vi "GetRange.vi"(11 "String":string) -> (0 "#Col Elements":i32, 1 "Start Column":i32, 2 "#RowElements":i32, 3 "Start Row":i32)   [LabVIEW 2014]
panel:
  # "Input"
  # "Output"
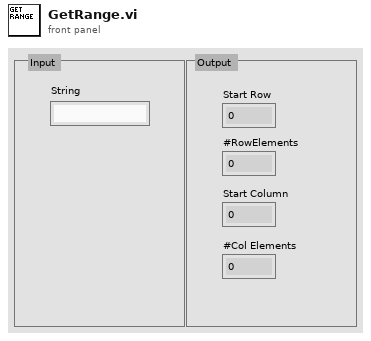
[diagram p1: front panel]
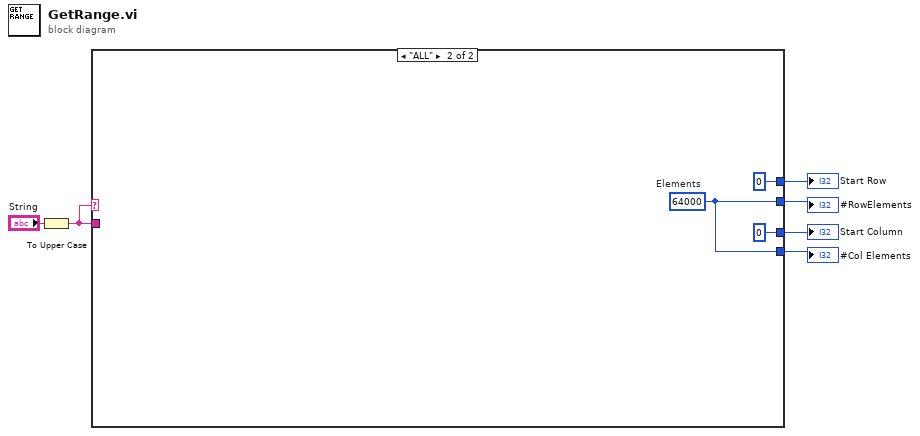
[diagram p0: block diagram]
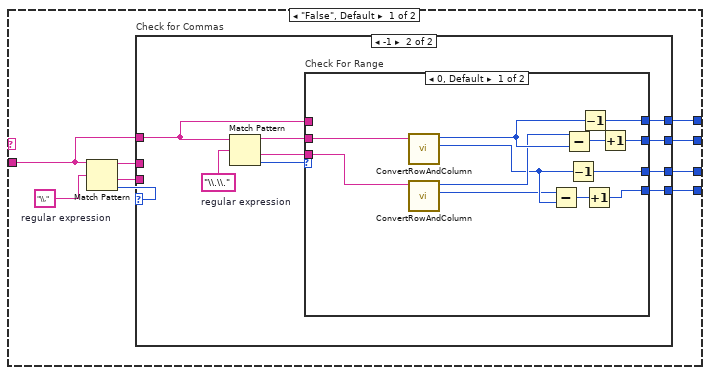
[diagram p2: hidden frame]
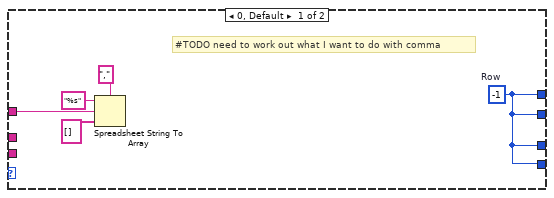
[diagram p3: hidden frame]
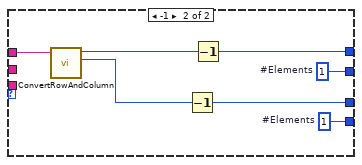
[diagram p4: hidden frame]
diagram:
  n1 = To Upper Case(1:"String") -> (0:w1:string)
  n2 = case shown="\"ALL\"" w1 {
    tunnel: [w11 0 ("Row")] -> w5
    tunnel: [w10 w49] -> w4
    tunnel: [w9 0 ("Row")] -> w3
    tunnel: [w8 w49] -> w2
    tunnel: w1 -> [w7 _]
    frame "False", Default {
      w12 = "\\,"  # regular expression
      n3 = Match Pattern(string=w7, regular expression=w12) -> (before substring=w14:string, after substring=w13:string, offset past match=w15:i32)  [unwired: 1 in, 1 out]
      n4 = case "Check for Commas" shown="-1" w15 {
        tunnel: w14 -> [_ _]
        tunnel: w13 -> [_ _]
        tunnel: w7 -> [w19 w25]
        tunnel: [w16 w24] -> w11
        tunnel: [w16 w23] -> w10
        tunnel: [w16 w22] -> w9
        tunnel: [w16 w21] -> w8
        frame 0, Default {
          w16 = -1  # Row
          # "#TODO need to work out what I want to do with comma"
          n5 = Spreadsheet String To Array(delimiter (Tab)=",", format string="%s", spreadsheet string=w19, array type (2D Dbl)=string[] []) -> ()  [unwired: 1 out]
        }
        frame -1 {
          w29 = "\\.\\."  # regular expression
          n6 = Match Pattern(string=w25, regular expression=w29) -> (before substring=w27:string, after substring=w26:string, offset past match=w28:i32)  [unwired: 1 in, 1 out]
          n7 = case "Check For Range" shown="0, Default" w28 {
            tunnel: w27 -> [w41 _]
            tunnel: w26 -> [w40 _]
            tunnel: w25 -> [_ w48]
            tunnel: [w31 w43] -> w24
            tunnel: [w32 w46] -> w23
            tunnel: [w30 w42] -> w22
            tunnel: [w33 w44] -> w21
            frame 0, Default {
              n8 = call "ConvertRowAndColumn.vi"("String"=w41) -> ("Column"=w35:i32, "Row"=w38:i32)  [unwired: 9 in]
              n9 = call "ConvertRowAndColumn.vi"("String"=w40) -> ("Column"=w34:i32, "Row"=w37:i32)  [unwired: 9 in]
              n10 = Subtract(x=w34, y=w35) -> (x-y=w39:i32)
              n11 = Subtract(x=w37, y=w38) -> (x-y=w36:i32)
              n12 = Decrement(x=w35) -> (x-1=w30:i32)
              n13 = Decrement(x=w38) -> (x-1=w31:i32)
              n14 = Increment(x=w39) -> (x+1=w33:i32)
              n15 = Increment(x=w36) -> (x+1=w32:i32)
            }
            frame -1 {
              w44 = 1  # #Elements
              w46 = 1  # #Elements
              n16 = call "ConvertRowAndColumn.vi"("String"=w48) -> ("Column"=w45:i32, "Row"=w47:i32)  [unwired: 9 in]
              n17 = Decrement(x=w45) -> (x-1=w42:i32)
              n18 = Decrement(x=w47) -> (x-1=w43:i32)
            }
          }
        }
      }
    }
    frame "ALL" {
      w49 = 64000  # Elements
    }
  }
  "Start Row" <- w5
  "#RowElements" <- w4
  "Start Column" <- w3
  "#Col Elements" <- w2
